vi "Movement Picture.vi"(5 "Spin or not to spin\n(add pause sign in corner if not spinning)":bool=TRUE, 6 "rect":T1={"left"=0, "top"=0, "right"=407, "bottom"=407}, 7 "Rotation Radius":dbl=50.0 format="%#_13g", 8 "Arrow Size":dbl=15.0 format="%#_13g", 9 "RightJoyStick X":dbl(slide) scale=-1.0..1.0, 10 "Y":dbl=0.007201, 11 "X":dbl=-0.002561) -> (3 "2D Picture":picture)   [LabVIEW 2017]
panel:
  out "output cluster 2":cluster{dbl, dbl}={149.4878, 198.5598}
  out "output cluster":cluster{dbl, dbl}={199.4878, 198.5598}
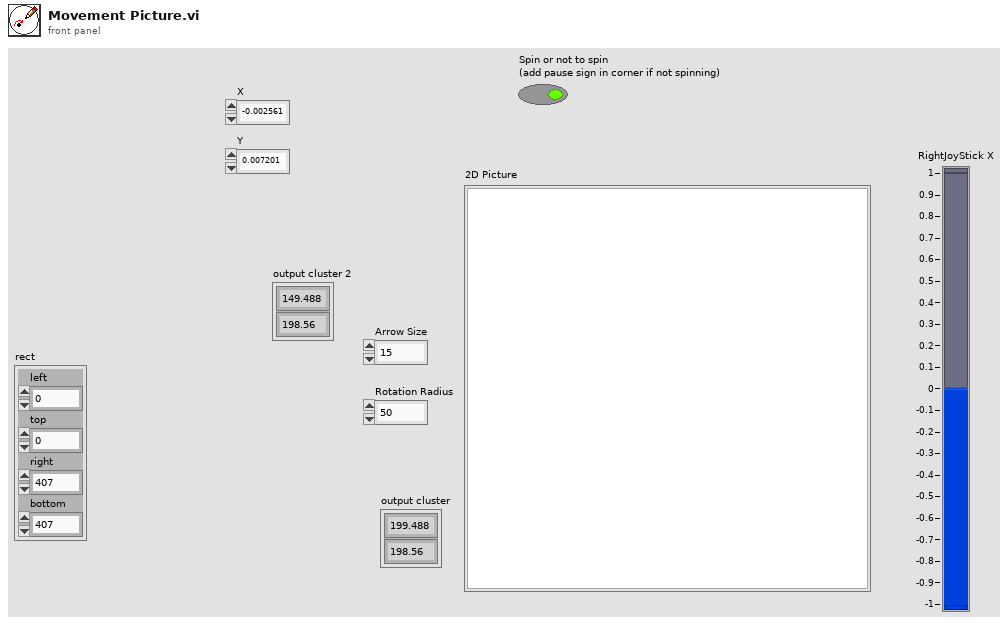
[diagram p1: front panel]
types:
  T1 = cluster{"left":i16, "top":i16, "right":i16, "bottom":i16}
  T2 = cluster{"Width":u16, "Style":enum32{"Solid", "Dash", "Dot", "DashDot", "DashDotDot"}}
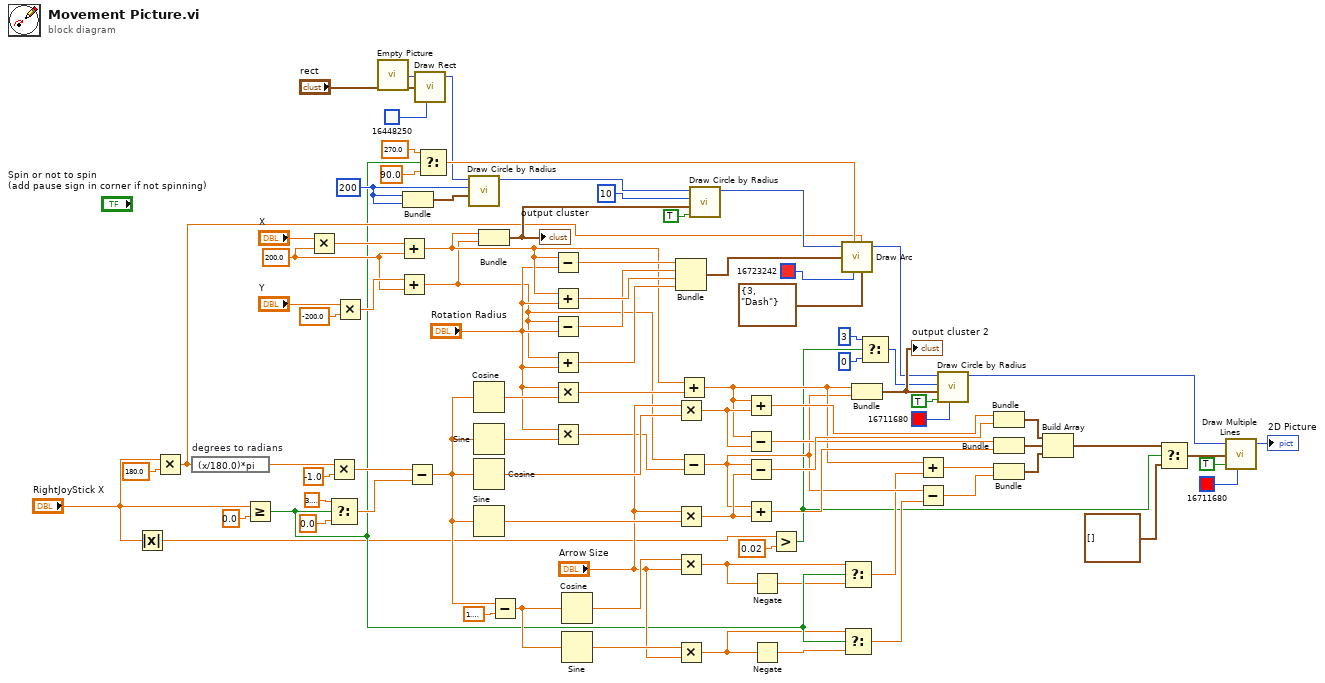
[diagram p0: block diagram]
diagram:
  w84 = 200.0 ("y")
  w89 = i16 200 ("radius")
  n1 = Absolute Value(x="RightJoyStick X") -> (abs(x)=w12:dbl)
  n2 = Multiply(x="RightJoyStick X", y=180.0) -> (x*y=w41:dbl)
  n3 = expression code="(x/180.0)*pi" "degrees to radians"(w41) -> (w36:dbl)
  n4 = Greater Or Equal?(x="RightJoyStick X", y=0.0) -> (x >= y?=w20:bool)
  n5 = Multiply(x="X", y=w84) -> (x*y=w87:dbl)
  n6 = Multiply(x=w36, y=-1.0) -> (x*y=w34:dbl)
  n7 = Select(t=3.141592653589793, s=w20, f=0.0) -> (s? t:f=w23:dbl)
  n8 = Multiply(x="Y", y=-200.0) -> (x*y=w86:dbl)
  n9 = call "Empty Picture"() -> ("empty picture"=w65:picture)
  n10 = Add(x=w87, y=w84) -> (x+y=w42:dbl)
  n11 = Add(x=w86, y=w84) -> (x+y=w33:dbl)
  n12 = Bundle("radius"=w89, "radius"=w89) -> (w88:cluster{"radius":i16, "radius":i16})  [unwired: 1 in]
  n13 = Subtract(x=w34, y=w23) -> (x-y=w24:dbl)
  n14 = call <vilib>:"Draw Rect.vi"("picture"=w65, "rect"="rect", "color(black)"=u32 16448250) -> ("new picture"=w66:picture)  [unwired: 6 in]
  n15 = Select(t=270.0, s=w20, f=90.0) -> (s? t:f=w75:dbl)
  n16 = call <vilib>:"Draw Circle by Radius.vi"("pixel center"=w88, "radius"=w89, "picture"=w66) -> ("new picture"=w83:picture)  [unwired: 8 in]
  n17 = Cosine(x=w24) -> (cos(x)=w40:dbl)
  n18 = Sine(x=w24) -> (sin(x)=w39:dbl)
  n19 = Cosine(x=w24) -> (cos(x)=w61:dbl)
  n20 = Sine(x=w24) -> (sin(x)=w55:dbl)
  n21 = Bundle(w42, w33) -> (w81:cluster{dbl, dbl})  [unwired: 1 in]
  "output cluster" <- w81
  n22 = Subtract(x=w24, y=1.5707963267948966) -> (x-y=w48:dbl)
  n23 = Subtract(x=w42, y="Rotation Radius") -> (x-y=w71:dbl)
  n24 = Add(x=w42, y="Rotation Radius") -> (x+y=w70:dbl)
  n25 = Subtract(x=w33, y="Rotation Radius") -> (x-y=w69:dbl)
  n26 = Add(x=w33, y="Rotation Radius") -> (x+y=w68:dbl)
  n27 = Multiply(x="Rotation Radius", y=w40) -> (x*y=w37:dbl)
  n28 = Multiply(x="Rotation Radius", y=w39) -> (x*y=w32:dbl)
  n29 = Cosine(x=w48) -> (cos(x)=w46:dbl)
  n30 = Sine(x=w48) -> (sin(x)=w47:dbl)
  n31 = Bundle(w71, w69, w70, w68) -> (w67:cluster{dbl, dbl, dbl, dbl})  [unwired: 1 in]
  n32 = Multiply(x="Arrow Size", y=w61) -> (x*y=w53:dbl)
  n33 = Multiply(x="Arrow Size", y=w55) -> (x*y=w50:dbl)
  n34 = Multiply(x=w46, y="Arrow Size") -> (x*y=w14:dbl)
  n35 = Multiply(x=w47, y="Arrow Size") -> (x*y=w18:dbl)
  n36 = Add(x=w42, y=w37) -> (x+y=w30:dbl)
  n37 = Subtract(x=w33, y=w32) -> (x-y=w29:dbl)
  n38 = call <vilib>:"Draw Circle by Radius.vi"("fill?(F)"=TRUE, "pixel center"=w81, "radius"=i16 10, "picture"=w83) -> ("new picture"=w79:picture)  [unwired: 7 in]
  n39 = Add(x=w30, y=w53) -> (x+y=w56:dbl)
  n40 = Subtract(x=w30, y=w53) -> (x-y=w52:dbl)
  n41 = Subtract(x=w29, y=w50) -> (x-y=w54:dbl)
  n42 = Add(x=w29, y=w50) -> (x+y=w51:dbl)
  n43 = Negate(x=w14) -> (-x=w15:dbl)
  n44 = Negate(x=w18) -> (-x=w19:dbl)
  n45 = Greater?(x=w12, y=0.02 ("f")) -> (0:w10:bool)
  n46 = call <vilib>:"Draw Arc.vi"("picture"=w79, "start angle[degrees]"=w75, "rect"=w67, "color(black)"=u32 16723242, "arc size[degrees]"=w41, "pen"=T2 {"Width"=3, "Style"=enum."Dash"}) -> ("new picture"=w26:picture)  [unwired: 3 in]
  n47 = Select(t=w14, s=w20, f=w15) -> (s? t:f=w16:dbl)
  n48 = Select(t=w18, s=w20, f=w19) -> (s? t:f=w17:dbl)
  n49 = Bundle(w30, w29) -> (w28:cluster{dbl, dbl})  [unwired: 1 in]
  "output cluster 2" <- w28
  n50 = Select(t=i16 3 ("radius"), s=w10, f=i16 0) -> (s? t:f=w6:i16)
  n51 = Add(x=w30, y=w16) -> (x+y=w43:dbl)
  n52 = Subtract(x=w29, y=w17) -> (x-y=w44:dbl)
  n53 = call <vilib>:"Draw Circle by Radius.vi"("color(black)"=u32 16711680, "fill?(F)"=TRUE, "pixel center"=w28, "radius"=w6, "picture"=w26) -> ("new picture"=w27:picture)  [unwired: 6 in]
  n54 = Bundle(w56, w54) -> (w59:cluster{dbl, dbl})  [unwired: 1 in]
  n55 = Bundle(w52, w51) -> (w58:cluster{dbl, dbl})  [unwired: 1 in]
  n56 = Bundle(w43, w44) -> (w57:cluster{dbl, dbl})  [unwired: 1 in]
  n57 = Build Array(w59, w58, w57) -> (w9:cluster{dbl, dbl}[])
  n58 = Select(t=w9, s=w10, f=cluster{"x":i16, "y":i16}[] [] ("line endpoints")) -> (s? t:f=w7:cluster{"x":dbl, "y":dbl}[])
  n59 = call <vilib>:"Draw Multiple Lines.vi"("picture"=w27, "line endpoints"=w7, "fill?(F)"=TRUE, "color(black)"=u32 16711680) -> ("new picture"=→"2D Picture":picture)  [unwired: 5 in]
